vi "alg_SVD (SubVI).vi"(0 "matrix":dbl[][](array[numeric]), 5 "only Specific?":bool=TRUE, 11 "에러 입력(에러 없음)":errorcluster) -> (3 "sv":dbl[](array[numeric]), 4 "참조 번호 출력":refnum<k35>, 6 "u":dbl[][](array[numeric]), 8 "s":dbl[][](array[numeric]), 10 "vh":dbl[][](array[numeric]), 15 "에러 출력":errorcluster)   [LabVIEW 2018]
uses:
  PythonConfigGlobal.vi
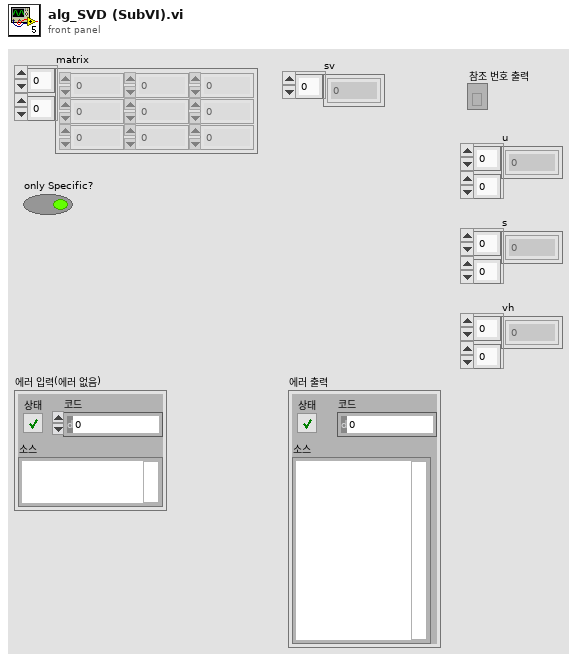
[diagram p1: front panel]
types:
  T1 = cluster{"sv":dbl[], "u":dbl[][], "s":dbl[][], "vh":dbl[][]}
  T2 = cluster{"session out":refnum<k35>, "appended path":path}
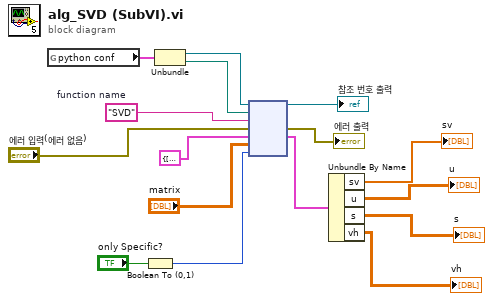
[diagram p0: block diagram]
diagram:
  w2 = "SVD"  # function name
  n1 = global read "PythonConfigGlobal.vi" "python conf"() -> (w5:T2)
  n2 = Boolean To (0,1)(Boolean="only Specific?") -> (0, 1=w8:i16)
  n3 = Unbundle(w5) -> ("session out"=w3:refnum<k35>, "appended path"=w4:path)
  n4 = node(w3, w4, w2, "에러 입력(에러 없음)", T1 {"sv"=[], "u"=[], "s"=[], "vh"=[]}, "matrix", w8) -> (→"참조 번호 출력":refnum<k35>, →"에러 출력":errorcluster, w12:T1)  [unwired: 2 in, 2 out]
  n5 = Unbundle By Name(w12) -> ("sv"=→"sv":dbl[], "u"=→"u":dbl[][], "s"=→"s":dbl[][], "vh"=→"vh":dbl[][])
